vi "Store Actor Core Ref.vi"(8 "error in (no error)":errorcluster, 11 "IViewable In":refnum<class "IViewable.lvclass">) -> (0 "error out":errorcluster, 3 "IViewable Out":refnum<class "IViewable.lvclass">)   [LabVIEW 2020, in "MVA Framework.lvlib" / "IViewable.lvlib" / "IViewable.lvclass"]
doc: "获取视图 Actor Core 引用"
uses:
  IViewable.lvclass
  IViewable.lvclass/IViewable.ctl
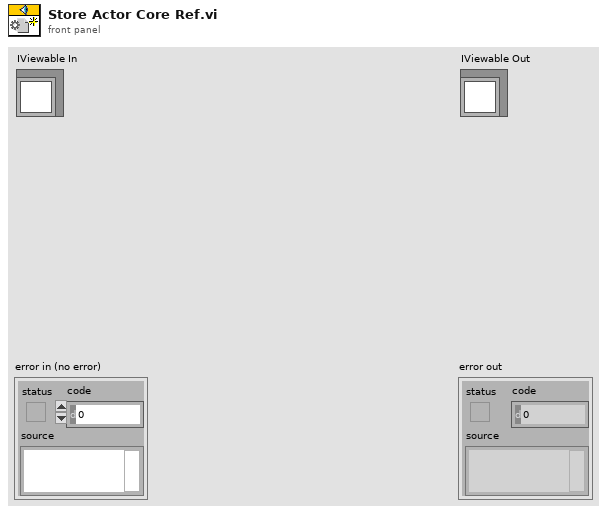
[diagram p1: front panel]
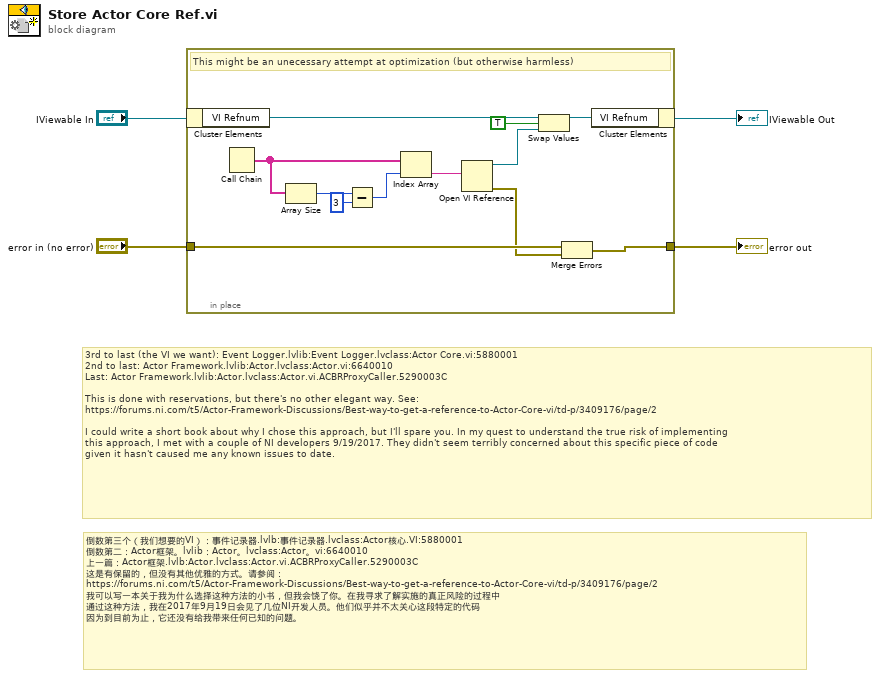
[diagram p0: block diagram]
diagram:
  # "倒数第三个（我们想要的VI）：事件记录器.lvlb:事件记录器.lvclass:Actor核心.VI:5880001\n倒数第二：Actor框架。lvlib：Actor。lvclass:Actor。vi:6640010\n上一篇：Actor框架.lvlb:Actor.lvclass:Actor.vi.ACBRProxyCaller.5290003C\n这是有保留的，但没有其他优雅的方式。请参阅：\nhttps://forums.ni.com/t5/Actor-Framework-Discussions/Best-way-to-get-a-reference-to-Actor-Core-vi/td-p/3409176/page/2\n我可以写一本关于我为什么选择这种方法的小书，但我会饶了你。在我寻求了解实施的真正风险的过程中\n通过这种方法，我在2017年9月19日会见了几位NI开发人员。他们似乎并不太关心这段特定的代码\n因为到目前为止，它还没有给我带来任何已知的问题。"
  # "3rd to last (the VI we want): Event Logger.lvlib:Event Logger.lvclass:Actor Core.vi:5880001\n2nd to last: Actor Framework.lvlib:Actor.lvclass:Actor.vi:6640010\nLast: Actor Framework.lvlib:Actor.lvclass:Actor.vi.ACBRProxyCaller.5290003C\n\nThis is done with reservations, but there's no other elegant way. See:\nhttps://forums.ni.com/t5/Actor-Framework-Discussions/Best-way-to-get-a-reference-to-Actor-Core-vi/td-p/3409176/page/2\n\nI could write a short book about why I chose this approach, but I'll spare you. In my quest to understand the true risk of implementing\nthis approach, I met with a couple of NI developers 9/19/2017. They didn't seem terribly concerned about this specific piece of code\ngiven it hasn't caused me any known issues to date."
  n1 = in-place {
    in-place-border: [w11] -> w4
    in-place-border: "error in (no error)" -> [w10]
    # "This might be an unecessary attempt at optimization (but otherwise harmless)"
    n2 = in-place-cluster #1("IViewable In") -> ("VI Refnum"=w8:refnum<vi>)
    n3 = Call Chain() -> (call chain=w14:string[])
    n4 = Array Size(array=w14) -> (size(s)=w16:i32)
    n5 = Subtract(x=w16, y=3) -> (x-y=w13:i32)
    n6 = Index Array(array=w14, index=w13) -> (element=w12:string)
    n7 = Open VI Reference(vi path=w12) -> (vi reference=w6:refnum<vi>, error out=w9:errorcluster)  [unwired: 5 in]
    n8 = Swap Values(12:w8, 13:TRUE ("?(T)"), 14:w6) -> (1:w7:refnum<vi>)  [unwired: 1 out]
    n9 = Merge Errors(w10, w9) -> (w11:errorcluster)
    n10 = in-place-cluster #1("VI Refnum"=w7) -> (→"IViewable Out":refnum<class "IViewable.lvclass">)
  }
  "error out" <- w4
